vi "Calculate Distance to Ball.vi"(6 "Ball Diameter (in)":dbl, 8 "results":T1, 10 "FOV (deg)":dbl, 11 "Image Src (in)":T2) -> (0 "output cluster":T1, 1 "Off Angle":dbl, 3 "Image Src (out)":T2, 4 "Distance":dbl)   [LabVIEW 2023]
uses:
  <vilib>/vision/Image Controls.llb/IMAQ Image.ctl
  Target Fields.ctl
  <vilib>/ptbypt/NI_PtbyPt.lvlib
panel:
  out "Raw Ball DIstance":dbl
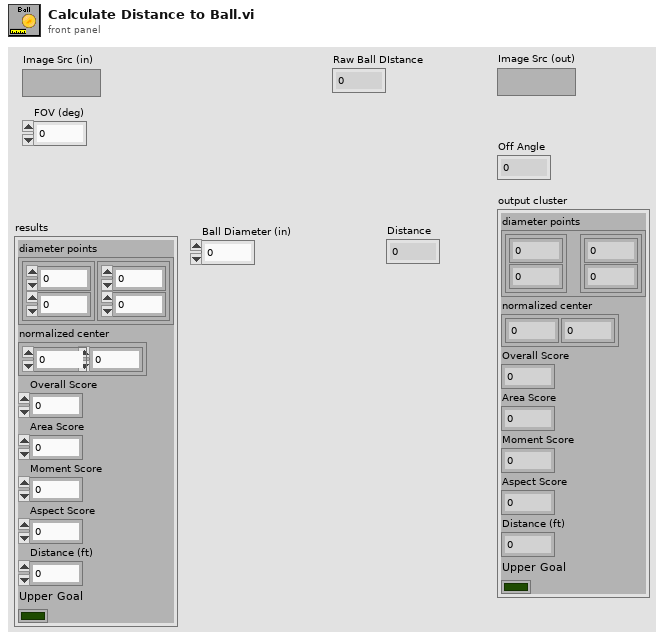
[diagram p1: front panel]
types:
  T1 = typedef "Target Fields.ctl" = cluster{"diameter points":cluster{"first point":cluster{"x":dbl, "y":dbl}, "projected point":cluster{"x":dbl, "y":dbl}}, "normalized center":cluster{"x":dbl, "y":dbl}, "Overall Score":dbl, "Area Score":dbl, "Moment Score":dbl, "Aspect Score":dbl, "Distance (ft)":dbl, "Upper Goal":bool}
  T2 = typedef "IMAQ Image.ctl" = refnum<image>
  T3 = cluster{"first point":cluster{"x":dbl, "y":dbl}, "projected point":cluster{"x":dbl, "y":dbl}}
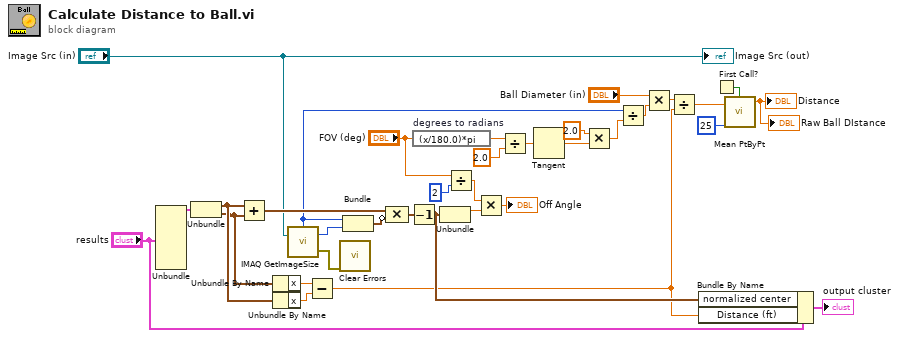
[diagram p0: block diagram]
diagram:
  n1 = Unbundle("results") -> ("diameter points"=w19:T3)  [unwired: 7 out]
  n2 = Unbundle(w19) -> ("first point"=w16:cluster{"x":dbl, "y":dbl}, "projected point"=w15:cluster{"x":dbl, "y":dbl})
  n3 = Add(x=w16, y=w15) -> (x+y=w23:cluster{"x":dbl, "y":dbl})
  n4 = Unbundle By Name(w15) -> ("x"=w14:dbl)
  n5 = Unbundle By Name(w16) -> ("x"=w13:dbl)
  n6 = call "IMAQ GetImageSize"("Image"="Image Src (in)") -> ("Y Resolution"=w22:i32, "X Resolution"=w11:i32, "error out"=w25:errorcluster)  [unwired: 3 in]
  n7 = Subtract(x=w14, y=w13) -> (x-y=w6:dbl)
  n8 = call <vilib>:"Clear Errors.vi"("error in (no error)"=w25) -> ()  [unwired: 5 in, 2 out]
  n9 = Bundle("X Resolution"=w11, "Y Resolution"=w22) -> (w24:cluster{"X Resolution":i32, "Y Resolution":i32})  [unwired: 1 in]
  n10 = Compound Arithmetic op=MULTIPLY(w23, invert w24) -> (w21:cluster{dbl, dbl})
  n11 = Decrement(x=w21) -> (x-1=w7:cluster{dbl, dbl})
  n12 = expression code="(x/180.0)*pi" "degrees to radians"("FOV (deg)") -> (w29:dbl)
  n13 = Unbundle(w7) -> (w10:dbl)  [unwired: 1 out]
  n14 = Divide(x="FOV (deg)", y=2) -> (x/y=w9:dbl)
  n15 = Multiply(x=w9, y=w10) -> (x*y=→"Off Angle":dbl)
  n16 = Divide(x=w29, y=2.0) -> (x/y=w33:dbl)
  n17 = Tangent(1:w33) -> (0:w32:dbl)
  n18 = Multiply(x=2.0, y=w32) -> (x*y=w30:dbl)
  n19 = Divide(x=w11, y=w30) -> (x/y=w27:dbl)
  n20 = Multiply(x="Ball Diameter (in)", y=w27) -> (x*y=w26:dbl)
  n21 = Divide(x=w26, y=w6) -> (x/y=w3:dbl)
  n22 = Bundle By Name(cluster="results", "normalized center"=w7, "Distance (ft)"=w6) -> (→"output cluster":T1)
  n23 = First Call?() -> (First Call?: T/F=w2:bool)
  n24 = call <vilib>:"Mean PtByPt.vi"("x"=w3, "sample length"=25, "initialize"=w2) -> ("mean"=→"Distance" →"Raw Ball DIstance":dbl)  [unwired: 1 in, 1 out]
  "Image Src (out)" <- "Image Src (in)"
